vi "LogData.vi"(8 "error in (no error)":errorcluster, 10 "Start time":u32, 11 "Refmum":refnum<file>) -> (0 "error out":errorcluster, 3 "Byte Stream File out":refnum<file>)   [LabVIEW 2017]
uses:
  DataNames.ctl
  LogOperation.ctl
  Framework/Robot Global Data.vi
  <vilib>/NI_Real-Time Target Support.lvlib
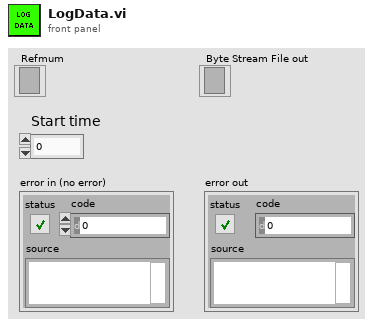
[diagram p1: front panel]
types:
  T1 = typedef "DataNames.ctl" = enum16{"RobotMode", "FMSConnected", "DriveLeft", "DriveRight", "EncoderLeft", "EncoderRight", "Angle", "LocationX", "LocationY", "CPU", "DriveOperation", "Battery"}
  T2 = typedef "LogOperation.ctl" = enum16{"Set", "Get All", "Init"}
  T3 = typedef "NI_Real-Time Target Support.lvlib/RT CPU Load.ctl" = cluster{"Total (%)":dbl, "Time Critical (%)":dbl, "Timed Structures (%)":dbl, "High (%)":dbl, "Above Normal (%)":dbl, "Normal (%)":dbl, "Background (%)":dbl, "Idle (%)":dbl, "ISR (%)":dbl}
  T4 = typedef "WPI_DriverStationRobotMode2.ctl" = enum16{"Autonomous Disabled", "Autonomous Enabled", "Teleop Disabled", "Teleop Enabled", "Disconnected", "Finish", "Test Disabled", "Test Enabled", "Emergency Stopped"}
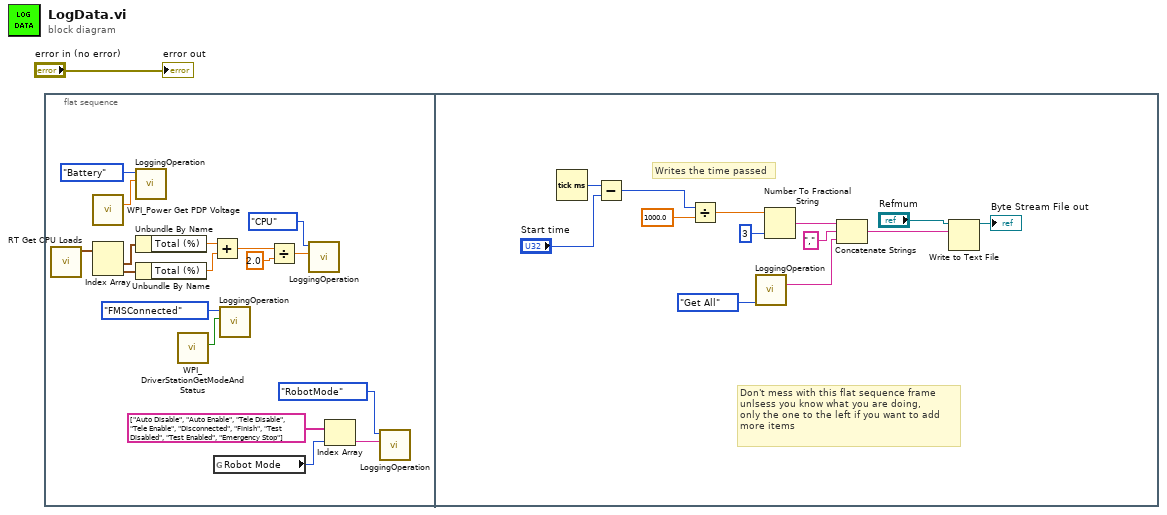
[diagram p0: block diagram]
diagram:
  n1 = flat-sequence {
    frame #0 {
      n2 = call <vilib>:"RT Get CPU Loads.vi"() -> ("CPU loads"=w16:T3[])  [unwired: 10 in, 1 out]
      n3 = call <vilib>:"WPI_Power Get PDP Voltage.vi"() -> ("voltage (V)"=w7:dbl)  [unwired: 14 in, 1 out]
      n4 = Index Array(array=w16) -> (element #1=w17:T3, element #2=w18:T3)  [unwired: 2 in]
      n5 = call "LoggingOperation.vi"("Data"=w7, "Name"=DataNames."Battery") -> ()  [unwired: 9 in, 1 out]
      n6 = Unbundle By Name(w17) -> ("Total (%)"=w5:dbl)
      n7 = Unbundle By Name(w18) -> ("Total (%)"=w6:dbl)
      n8 = call <vilib>:"WPI_DriverStationGetModeAndStatus.vi"() -> ("FMS Attached"=w14:bool)  [unwired: 10 in, 1 out]
      n9 = Add(x=w5, y=w6) -> (x+y=w4:dbl)
      n10 = global read "Robot Global Data.vi" "Robot Mode"() -> (w13:T4)
      n11 = call "LoggingOperation.vi"("Data"=w14, "Name"=DataNames."FMSConnected") -> ()  [unwired: 9 in, 1 out]
      n12 = Divide(x=w4, y=2.0) -> (x/y=w2:dbl)
      n13 = call "LoggingOperation.vi"("Data"=w2, "Name"=DataNames."CPU") -> ()  [unwired: 9 in, 1 out]
      n14 = Index Array(array=string[] ["Auto Disable", "Auto Enable", "Tele Disable", "Tele Enable", "Disconnected", "Finish", "Test Disabled", "Test Enabled", "Emergency Stop"], index=w13) -> (element=w15:string)
      n15 = call "LoggingOperation.vi"("Data"=w15, "Name"=DataNames."RobotMode") -> ()  [unwired: 9 in, 1 out]
    }
    frame #1 {
      # "Don't mess with this flat sequence frame\nunlsess you know what you are doing,\nonly the one to the left if you want to add\nmore items"
      # "Writes the time passed"
      n16 = Tick Count (ms)() -> (millisecond timer value=w31:u32)
      n17 = Subtract(x=w31, y="Start time") -> (x-y=w29:u32)
      n18 = Divide(x=w29, y=1000.0 ("input 9")) -> (x/y=w24:dbl)
      n19 = call "LoggingOperation.vi"("Operation"=LogOperation."Get All") -> ("Log String"=w20:string)  [unwired: 10 in]
      n20 = Number To Fractional String(number=w24, precision (6)=i16 3) -> (F-format string=w22:string)  [unwired: 2 in]
      n21 = Concatenate Strings(w22, "," ("string"), w20) -> (w19:string)
      n22 = Write to Text File(file (use dialog)="Refmum", text=w19) -> (refnum out=→"Byte Stream File out":refnum<file>)  [unwired: 2 in, 2 out]
    }
  }
  "error out" <- "error in (no error)"
